vi "Write Branch Name.vi"(8 "error in":errorcluster, 10 "Name":string, 11 "Tree in":refnum<class "Tree.lvclass">) -> (0 "error out":errorcluster, 3 "Tree out":refnum<class "Tree.lvclass">)   [LabVIEW 2019, in "Tree.lvclass"]
uses:
  Tree.lvclass
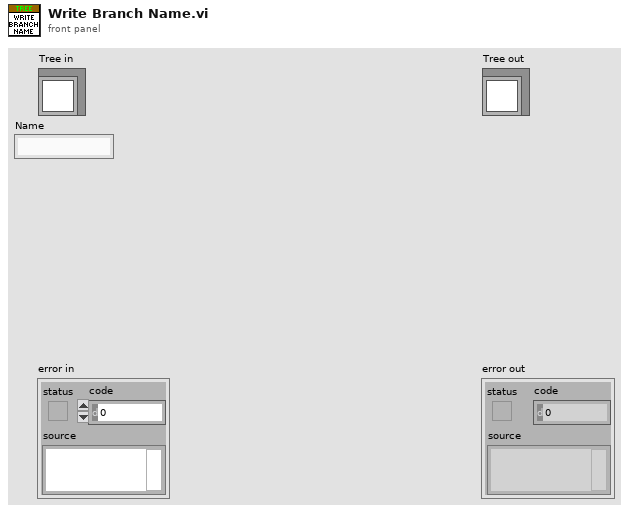
[diagram p1: front panel]
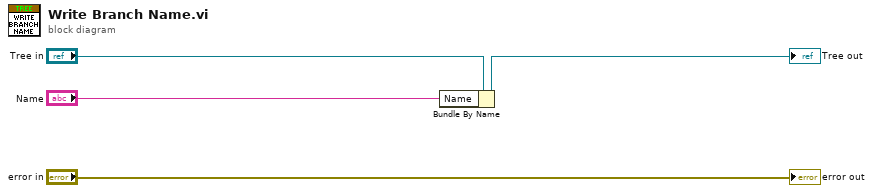
[diagram p0: block diagram]
diagram:
  n1 = Bundle By Name(cluster="Tree in", "Name"="Name") -> (→"Tree out":refnum<class "Tree.lvclass">)
  "error out" <- "error in"
